vi "PID Control Input Filter (DBL Array).vi"(3 "reinitialize? (F)":bool, 4 "input":dbl[](array[numeric])=[0.0] format="%.2f") -> (1 "output":dbl[](array[numeric]) format="%.2f")   [LabVIEW 2020, in "NI_PID_pid.lvlib"]
doc: "Applies a fifth-order lowpass finite impulse response (FIR) filter to the input value. Filter cut-off frequency is designed to be 1/10 of the sample frequency of the input value. Use this VI to filter measured values, such as the process variable, in control applications. Use the DBL instance of this VI to implement a single control loop. Use the DBL Array instance to implement parallel multi-loop control."
uses:
  <vilib>/addons/control/pid/NI_PID_pid.lvlib
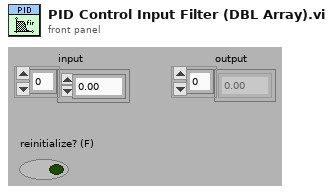
[diagram p1: front panel]
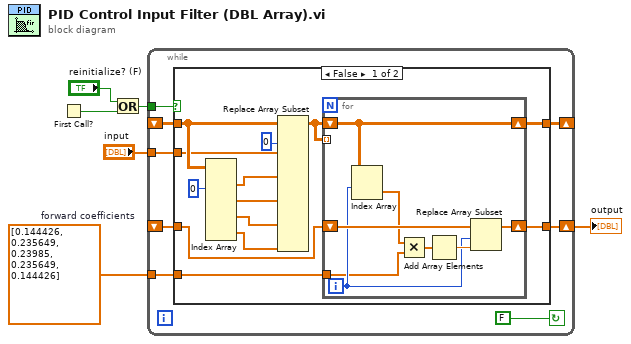
[diagram p0: block diagram]
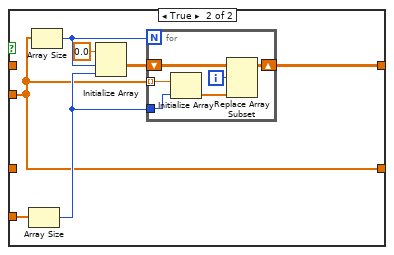
[diagram p2: hidden frame]
diagram:
  w5 = dbl[] [0.144426, 0.235649, 0.23985, 0.235649, 0.144426]  # forward coefficients
  n1 = First Call?() -> (First Call?: T/F=w1:bool)
  n2 = Or(x="reinitialize? (F)", y=w1) -> (x .or. y?=w6:bool)
  n3 = while {
    shift-left: _ -> [w10]
    shift-right: [w9] -> _
    tunnel: w6 -> [w11]
    tunnel: w5 -> [w12]
    tunnel: "input" -> [w14]
    shift-right: [w13] -> w3
    shift-left: _ -> [w7]
    stop <- FALSE continue-if-true
    n4 = case shown="False" w11 {
      tunnel: w12 -> [w18 w39]
      tunnel: w10 -> [w25 _]
      tunnel: [w27 w37] -> w13
      tunnel: [w16 w38] -> w9
      tunnel: w14 -> [w24 w37]
      tunnel: w7 -> [w17 _]
      frame False {
        n5 = Index Array(array=w25, index (col) #1=0 ("Disabled Index (col)")) -> (element #1=w22:dbl[], element #2=w21:dbl[], element #3=w20:dbl[], element #4=w19:dbl[])  [unwired: 7 in]
        n6 = Replace Array Subset(array=w25, new element #1=w24, index (col) #1=0 ("Disabled Index (col)"), new element #2=w22, new element #3=w21, new element #4=w20, new element #5=w19) -> (w15:dbl[][])  [unwired: 9 in]
        n7 = for {
          shift-right: [w32] -> w27
          shift-left: w17 -> [w34]
          tunnel: w18 -> [w28]
          shift-right: [w30] -> w16
          shift-left: w15 -> [w30]
          tunnel: w15 -> [_] mode=indexing
          i -> [w31]
          n8 = Index Array(array=w30, index (row)=w31) -> (element=w29:dbl[])  [unwired: 1 in]
          n9 = Multiply(x=w29, y=w28) -> (x*y=w35:dbl[])
          n10 = Add Array Elements(numeric array=w35) -> (sum=w33:dbl)
          n11 = Replace Array Subset(array=w34, new element=w33, index=w31) -> (w32:dbl[])
        }
      }
      frame True {
        n12 = Array Size(array=w39) -> (size(s)=w42:i32)
        n13 = Array Size(array=w37) -> (size(s)=w36:i32)
        n14 = Initialize Array(0.0 ("element"), w36, w42) -> (w41:dbl[][])
        n15 = for {
          N: w36 -> [_]
          tunnel: w42 -> [w48]
          shift-right: [w44] -> w38
          shift-left: w41 -> [w46]
          tunnel: w37 -> [w47] mode=indexing
          i -> [w43]
          n16 = Initialize Array(w47, w48) -> (w45:dbl[])
          n17 = Replace Array Subset(array=w46, new element=w45, index (row)=w43) -> (w44:dbl[][])  [unwired: 1 in]
        }
      }
    }
  }
  "output" <- w3
